vi "vi打开一个外部文件.vi"() -> ()   [LabVIEW 2010]
panel:
  in  "停止":bool
  in  "打开ppt":bool
  in  "打开word":bool
  in  "打开txt":bool
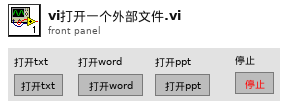
[diagram p1: front panel]
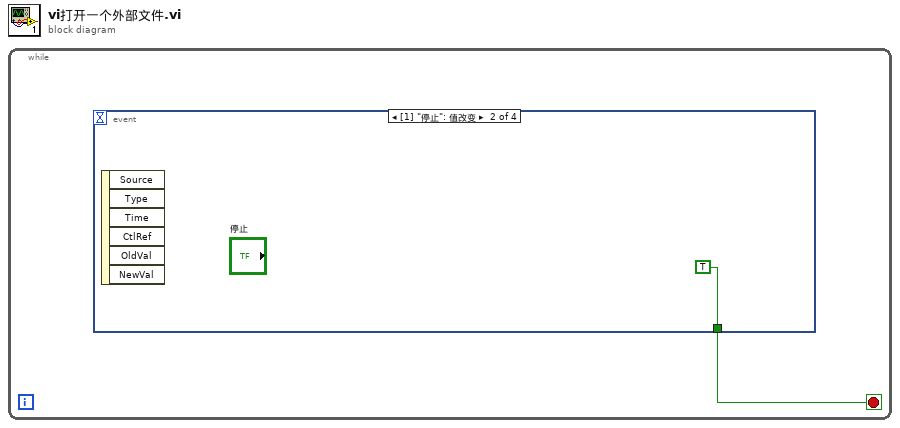
[diagram p0: block diagram]
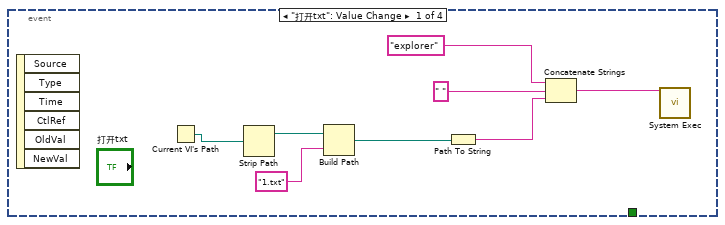
[diagram p2: hidden frame]
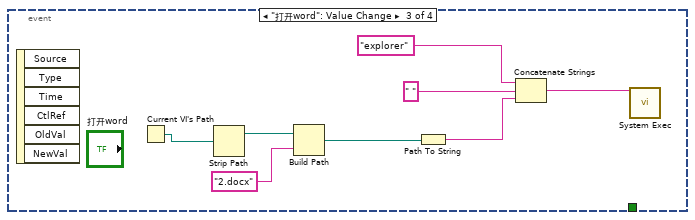
[diagram p3: hidden frame]
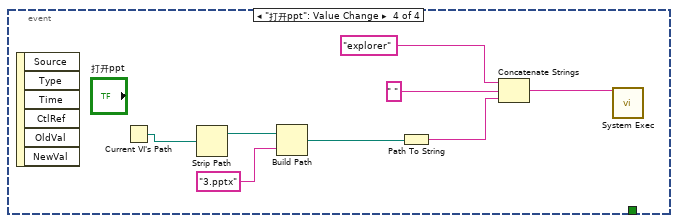
[diagram p4: hidden frame]
diagram:
  n1 = while {
    stop <- w1 stop-if-true
    n2 = event shown="[1] \"停止\": 值改变" {
      selector: _ -> [_ _ _ _]
      dyn-events: _ -> [_ _ _ _]
      timeout: _ -> [_ _ _ _]
      tunnel: [_ TRUE _ _] -> w1
      event "打开txt": Value Change {
        n3 = event-data() -> ()  [unwired: 1 in, 6 out]
        n4 = Current VI's Path() -> (path=w2:path)
        n5 = Strip Path(path=w2) -> (stripped path=w7:path)  [unwired: 1 out]
        n6 = Build Path(base path=w7, name or relative path="1.txt" ("名称或相对路径")) -> (appended path=w9:path)
        n7 = Path To String(path=w9) -> (string=w5:string)
        n8 = Concatenate Strings("explorer" ("字符串"), " " ("字符串"), w5) -> (w4:string)
        n9 = call <vilib>:"System Exec.vi"("command line"=w4) -> ()  [unwired: 7 in, 4 out]
      }
      event "停止": Value Change {
        n10 = event-data() -> ()  [unwired: 1 in, 6 out]
      }
      event "打开word": Value Change {
        n11 = event-data() -> ()  [unwired: 1 in, 6 out]
        n12 = Current VI's Path() -> (path=w11:path)
        n13 = Strip Path(path=w11) -> (stripped path=w16:path)  [unwired: 1 out]
        n14 = Build Path(base path=w16, name or relative path="2.docx" ("名称或相对路径")) -> (appended path=w18:path)
        n15 = Path To String(path=w18) -> (string=w14:string)
        n16 = Concatenate Strings("explorer" ("字符串"), " " ("字符串"), w14) -> (w13:string)
        n17 = call <vilib>:"System Exec.vi"("command line"=w13) -> ()  [unwired: 7 in, 4 out]
      }
      event "打开ppt": Value Change {
        n18 = event-data() -> ()  [unwired: 1 in, 6 out]
        n19 = Current VI's Path() -> (path=w19:path)
        n20 = Strip Path(path=w19) -> (stripped path=w24:path)  [unwired: 1 out]
        n21 = Build Path(base path=w24, name or relative path="3.pptx" ("名称或相对路径")) -> (appended path=w26:path)
        n22 = Path To String(path=w26) -> (string=w22:string)
        n23 = Concatenate Strings("explorer" ("字符串"), " " ("字符串"), w22) -> (w21:string)
        n24 = call <vilib>:"System Exec.vi"("command line"=w21) -> ()  [unwired: 7 in, 4 out]
      }
    }
  }
